vi "SetSimulationParameterDataStructure.vi"(8 "error in (no error)":errorcluster, 11 "SimulationParameter in":refnum<class "SimulationParameter.lvclass">) -> (0 "error out":errorcluster, 3 "SimulationParameter out":refnum<class "SimulationParameter.lvclass">)   [LabVIEW 2017, in "SimulationParameter.lvclass"]
uses:
  SimulationParameter.lvclass
  SimulationParameter.lvclass/SimulationParameter.ctl
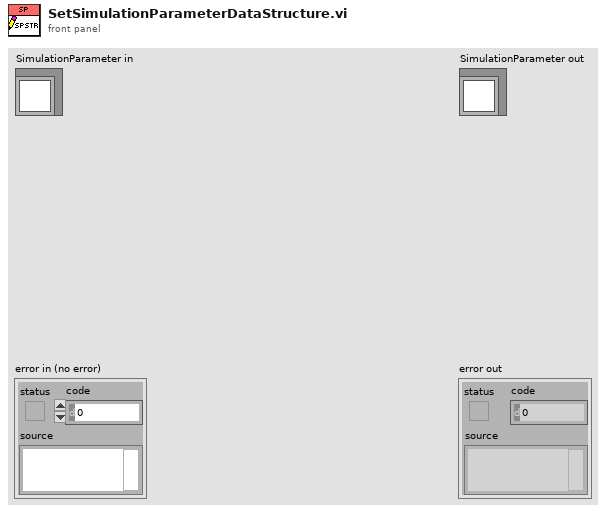
[diagram p1: front panel]
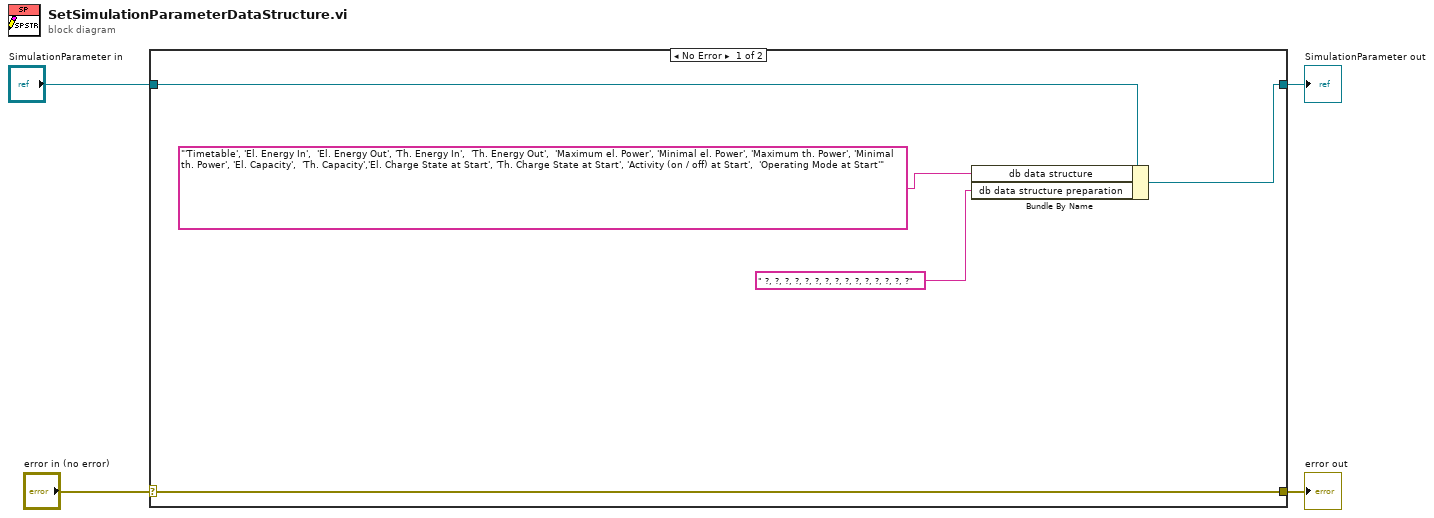
[diagram p0: block diagram]
diagram:
  n1 = case shown="No Error" "error in (no error)" {
    selector: "error in (no error)" -> [w9 w10]
    tunnel: [w9 w10] -> w3
    tunnel: [w7 w11] -> w1
    tunnel: "SimulationParameter in" -> [w8 w11]
    frame No Error {
      n2 = Bundle By Name(cluster=w8, "db data structure"="'Timetable', 'El. Energy In',  'El. Energy Out', 'Th. Energy In',  'Th. Energy Out',  'Maximum el. Power', 'Minimal el. Power', 'Maximum th. Power', 'Minimal th. Power', 'El. Capacity',  'Th. Capacity','El. Charge State at Start', 'Th. Charge State at Start', 'Activity (on / off) at Start',  'Operating Mode at Start'" ("string"), "db data structure preparation"=" ?, ?, ?, ?, ?, ?, ?, ?, ?, ?, ?, ?, ?, ?, ?") -> (w7:refnum<class "SimulationParameter.lvclass">)
    }
    frame Error {
    }
  }
  "error out" <- w3
  "SimulationParameter out" <- w1
